vi "Col_Velocity(Subvi).vi"(8 "Fs":dbl=110000.0 format="%#_13g", 9 "거리":dbl format="%#_13g", 10 "Station_index_2":i32, 11 "Station_index_1":i32) -> (0 "Averange_SoundSpeed":dbl, 2 "Water_Velocity":dbl)   [LabVIEW 2024]
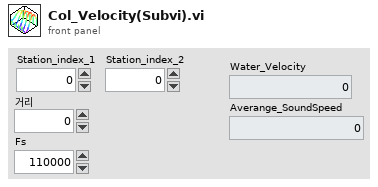
[diagram p1: front panel]
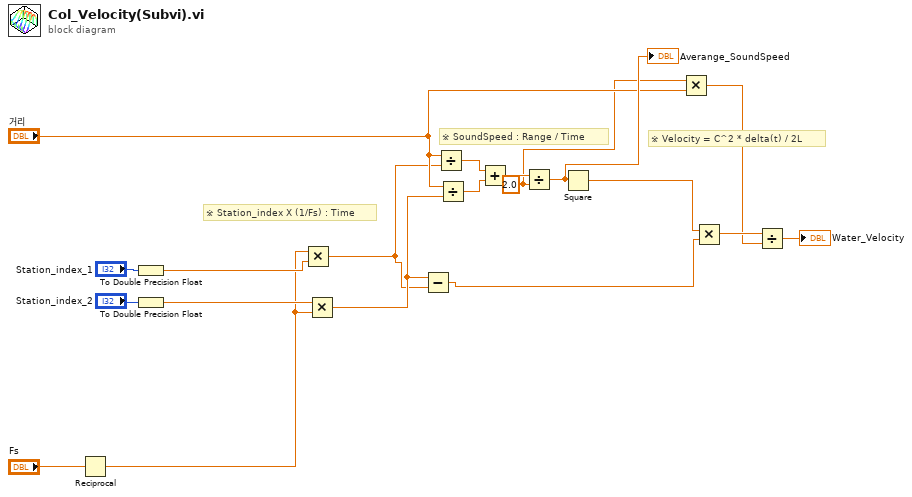
[diagram p0: block diagram]
diagram:
  w7 = 2.0 ("y")
  # "※ Velocity = C^2 * delta(t) / 2L"
  # "※ SoundSpeed : Range / Time"
  # "※ Station_index X (1/Fs) : Time"
  n1 = Reciprocal(x="Fs") -> (1/x=w4:dbl)
  n2 = To Double Precision Float(number="Station_index_1") -> (double precision float=w17:dbl)
  n3 = To Double Precision Float(number="Station_index_2") -> (double precision float=w16:dbl)
  n4 = Multiply(x=w4, y=w17) -> (x*y=w1:dbl)
  n5 = Multiply(x=w16, y=w4) -> (x*y=w2:dbl)
  n6 = Subtract(x=w2, y=w1) -> (x-y=w3:dbl)
  n7 = Divide(x="거리", y=w1) -> (x/y=w15:dbl)
  n8 = Divide(x="거리", y=w2) -> (x/y=w14:dbl)
  n9 = Add(x=w15, y=w14) -> (x+y=w13:dbl)
  n10 = Divide(x=w13, y=w7) -> (x/y=w12:dbl)
  "Averange_SoundSpeed" <- w12
  n11 = Square(x=w12) -> (x^2=w11:dbl)
  n12 = Multiply(x=w7, y="거리") -> (x*y=w9:dbl)
  n13 = Multiply(x=w11, y=w3) -> (x*y=w10:dbl)
  n14 = Divide(x=w10, y=w9) -> (x/y=→"Water_Velocity":dbl)
